vi "Computer Listener - Observed.vi"() -> ()   [LabVIEW 2025]
uses:
  Listener State.ctl
panel:
  out "Facilitator Address":string
  in  "Name ID":string
  out "Status":string
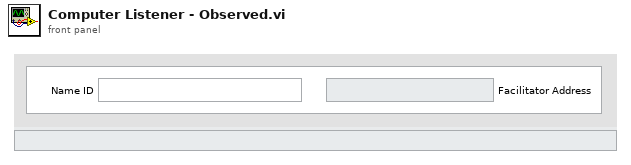
[diagram p1: front panel]
types:
  T1 = typedef "Listener State.ctl" = enum16{"Wait For Connection", "Send Response", "Wait For Another Query"}
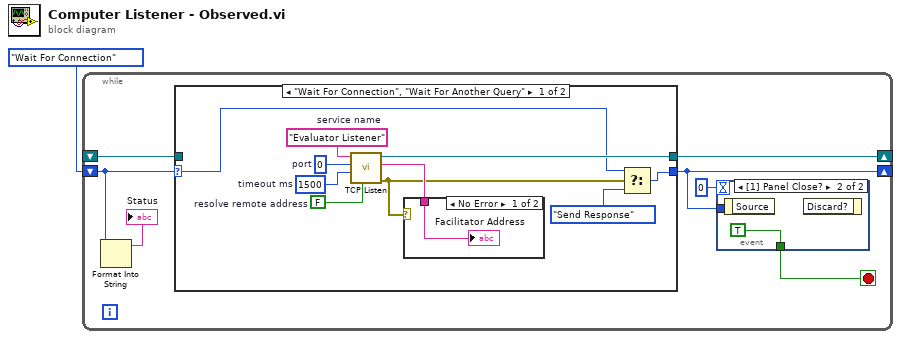
[diagram p0: block diagram]
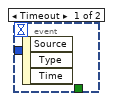
[diagram p2: hidden frame]
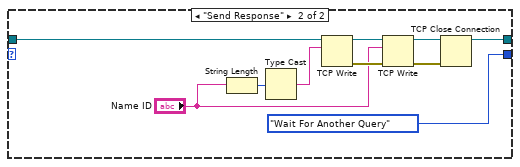
[diagram p4: hidden frame]
diagram:
  n1 = while {
    shift-right: [w8] -> _
    shift-left: _ -> [w7]
    shift-right: [w4] -> _
    shift-left: Listener_State."Wait For Connection" -> [w6]
    stop <- w2 stop-if-true
    n2 = Format Into String(w6) -> (resulting string=→"Status":string)  [unwired: 3 in, 1 out]
    n3 = case shown="\"Wait For Connection\", \"Wait For Another Query\"" w6 {
      selector: w6 -> [w13 _]
      tunnel: [w15 w22] -> w8
      tunnel: w7 -> [_ w23]
      tunnel: [w12 Listener_State."Wait For Another Query"] -> w4
      frame "Wait For Connection", "Wait For Another Query" {
        w14 = 1500  # timeout ms
        w17 = u16 0  # port
        w18 = "Evaluator Listener"  # service name
        w19 = FALSE  # resolve remote address
        n4 = call <vilib>:"TCP Listen.vi"("resolve remote address (T)"=w19, "timeout ms (wait forever: -1)"=w14, "port"=w17, "service name"=w18) -> ("error out"=w10:errorcluster, "remote address"=w16:string, "connection ID"=w15:refnum<k5>)  [unwired: 3 in, 2 out]
        n5 = case shown="No Error" w10 {
          tunnel: w16 -> [w20 _]
          frame No Error {
            "Facilitator Address" <- w20
          }
          frame Error {
          }
        }
        n6 = Select(t=w13, s=w10, f=Listener_State."Send Response") -> (s? t:f=w12:T1)
      }
      frame "Send Response" {
        n7 = String Length(string="Name ID") -> (length=w25:i32)
        n8 = Type Cast(x=w25) -> (*(type *) &x=w26:string)  [unwired: 1 in]
        n9 = TCP Write(connection ID=w23, data in=w26) -> (connection ID out=w27:refnum<k5>, error out=w28:errorcluster)  [unwired: 2 in, 1 out]
        n10 = TCP Write(connection ID=w27, data in="Name ID", error in (no error)=w28) -> (connection ID out=w30:refnum<k5>, error out=w29:errorcluster)  [unwired: 1 in, 1 out]
        n11 = TCP Close Connection(connection ID=w30, error in (no error)=w29) -> (connection ID out=w22:refnum<k5>)  [unwired: 1 in, 1 out]
      }
    }
    n12 = event shown="[1] Panel Close?" {
      selector: _ -> [_ _]
      dyn-events: _ -> [_ _]
      timeout: 0 -> [_ _]
      tunnel: w4 -> [_ _]
      tunnel: [_ TRUE] -> w2
      event Timeout {
        n13 = event-data() -> ()  [unwired: 1 in, 3 out]
      }
      event Panel Close? {
        n14 = event-data() -> ()  [unwired: 1 in, 1 out]
        n15 = event-data() -> ()  [unwired: 2 in, 1 out]
      }
    }
  }
